vi "DllFxpIntAccumulator_Int.vi"(6 "enable":bool, 8 "cinNbin":bool, 9 "isSub":bool, 10 "load":bool, 11 "x":i8) -> (2 "coutNbout":bool, 3 "sum":fxp<+,32,32>)   [LabVIEW 2017]
uses:
  <vilib>/rvi/FXPMathLib/basic elements/FxpIntAccumulator/subVIs/nifxpmath_IntAccumulator_SimConfig.ctl
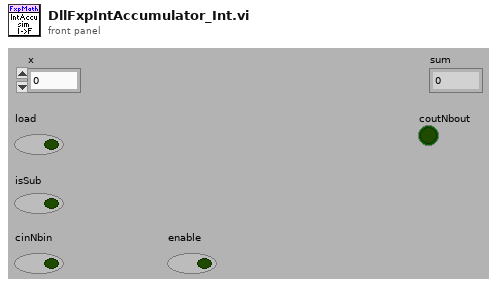
[diagram p1: front panel]
types:
  T1 = typedef "nifxpmath_IntAccumulator_SimConfig.ctl" = cluster{"kWordLengthIn":u16, "kWordLengthOut":u16, "kPrescaling":u16, "kNumOfCh":u16, "kIsSigned":bool, "kIsRegOut":bool}
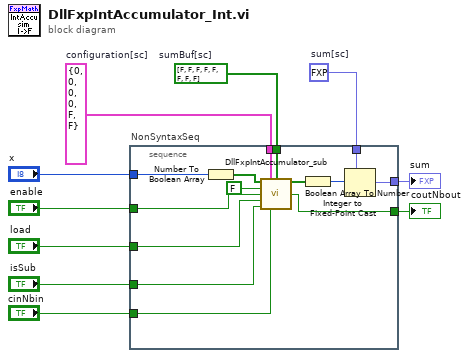
[diagram p0: block diagram]
diagram:
  w1 = T1 {"kWordLengthIn"=0, "kWordLengthOut"=0, "kPrescaling"=0, "kNumOfCh"=0, "kIsSigned"=FALSE, "kIsRegOut"=FALSE}  # configuration[sc]
  w5 = fxp<+,32,32> 0.0  # sum[sc]
  w3 = bool[] [FALSE, FALSE, FALSE, FALSE, FALSE, FALSE, FALSE, FALSE]  # sumBuf[sc]
  n1 = stacked-sequence "NonSyntaxSeq" {
    tunnel: [w24] -> w9
    tunnel: "load" -> [w19]
    tunnel: "enable" -> [w20]
    tunnel: w1 -> [w23]
    tunnel: "cinNbin" -> [w17]
    tunnel: "isSub" -> [w18]
    tunnel: "x" -> [w16]
    tunnel: w5 -> [w11]
    tunnel: [w12] -> w4
    tunnel: w3 -> [w22]
    frame #0 {
      n2 = Number To Boolean Array(number=w16) -> (Boolean array=w21:bool[])
      n3 = call <vilib>:"DllFxpIntAccumulator_sub.vi"("x"=w21, "configuration[sc]"=w23, "sumBuf[sc]"=w22, "xov"=FALSE, "enable"=w20, "load"=w19, "isSub"=w18, "cinNbin"=w17) -> ("s"=w13:bool[], "coutNbout"=w24:bool)  [unwired: 1 in, 5 out]
      n4 = Boolean Array To Number(Boolean array=w13) -> (number=w14:u64)
      n5 = Integer to Fixed-Point Cast(fixed-point type=w11, integer=w14) -> (fixed-point=w12:fxp<+,32,32>)
    }
  }
  "coutNbout" <- w9
  "sum" <- w4
